vi "UTIL Probe Reference.vi"(8 "error in (no error)":errorcluster, 11 "niDTS Comm EXE in":refnum<class "niDTS Comm EXE.lvclass">) -> (0 "error out":errorcluster, 2 "VI Refnum":refnum<vi>, 3 "niDTS Comm EXE out":refnum<class "niDTS Comm EXE.lvclass">)   [LabVIEW 2015, in "niDTS CommLib.lvlib" / "niDTS Comm EXE.lvclass"]
uses:
  niDTS Comm EXE.lvclass
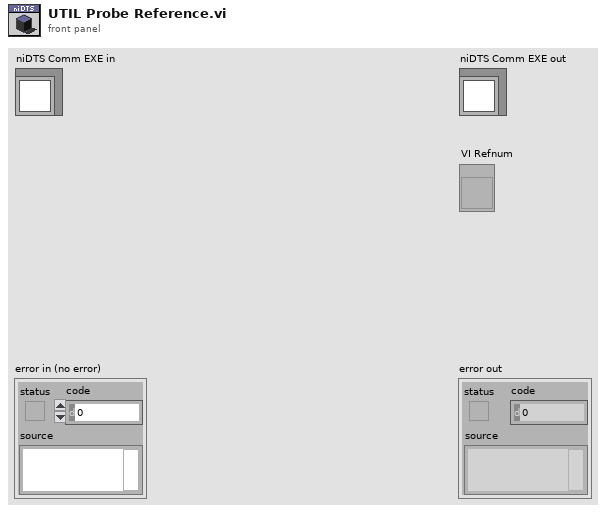
[diagram p1: front panel]
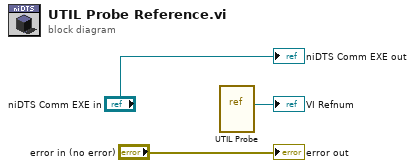
[diagram p0: block diagram]
diagram:
  n1 = vi-ref "UTIL Probe.vi"() -> (→"VI Refnum":refnum<vi>)
  "error out" <- "error in (no error)"
  "niDTS Comm EXE out" <- "niDTS Comm EXE in"
